vi "MTM2_issueCommand_switchForceBalanceSystem.vi"(8 "error in (no error)":errorcluster, 11 "command_switchForceBalanceSystem_Ctl":T1) -> (0 "error out":errorcluster, 2 "function return":i32, 3 "command_switchForceBalanceSystem_Ctl out":T1)   [LabVIEW 2018, in "SALLV_MTM2.lvlib"]
doc: "int MTM2_shm_issueCommand_switchForceBalanceSystemLV(MTM2_command_switchForceBalanceSystemLV *command_switchForceBalanceSystem_Ctl );"
uses:
  DataTypes/command_switchForceBalanceSystem.ctl
  SALLV_MTM2.lvlib
  SALLV_MTM2.so
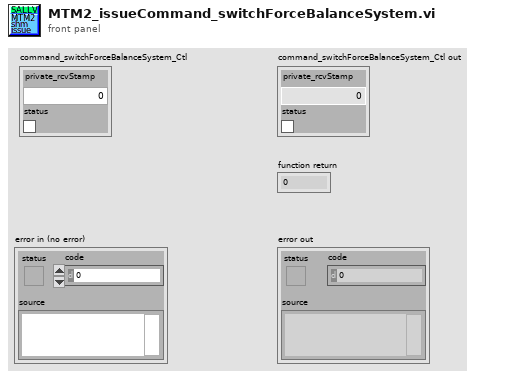
[diagram p1: front panel]
types:
  T1 = typedef "SALLV_MTM2.lvlib/command_switchForceBalanceSystem.ctl" = cluster{"private_rcvStamp":dbl, "status":bool}
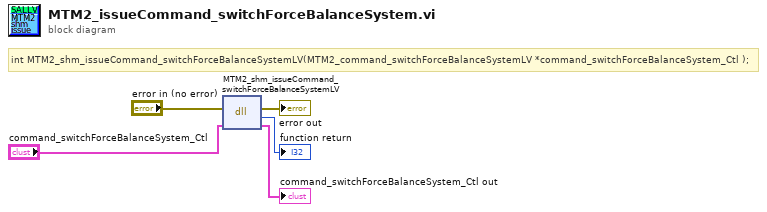
[diagram p0: block diagram]
diagram:
  # "int MTM2_shm_issueCommand_switchForceBalanceSystemLV(MTM2_command_switchForceBalanceSystemLV *command_switchForceBalanceSystem_Ctl );"
  n1 = dll-call lib="home/ttsai/Documents/salLabviewApi/SALLV_MTM2/SALLV_MTM2.*" fn="MTM2_shm_issueCommand_switchForceBalanceSystemLV"(error in="error in (no error)", "command_switchForceBalanceSystem_Ctl"="command_switchForceBalanceSystem_Ctl") -> (error out=→"error out":errorcluster, →"function return":i32, "command_switchForceBalanceSystem_Ctl"=→"command_switchForceBalanceSystem_Ctl out":T1)  [unwired: 2 in, 1 out]
